vi "SimpleNotifier.vi"() -> ()   [LabVIEW 2014]
panel:
  out "L2":i32
  out "L1":i32
  out "Data 2":dbl(graph)
  out "Data 1":dbl(graph)
  in  "Stop":bool
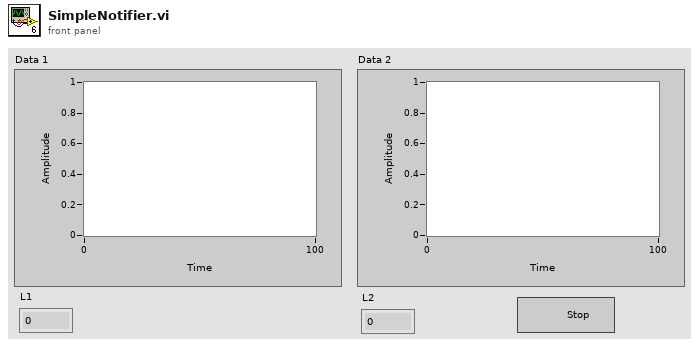
[diagram p1: front panel]
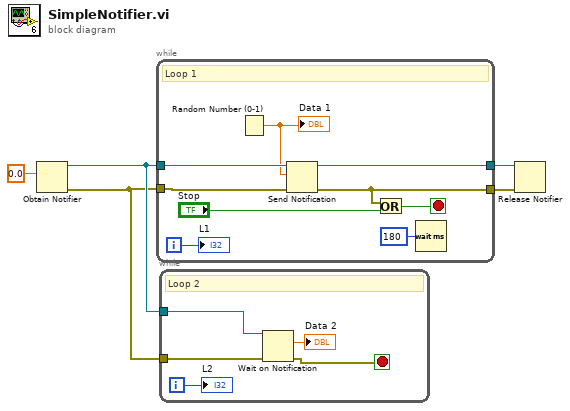
[diagram p0: block diagram]
diagram:
  n1 = Obtain Notifier(notification data type=0.0) -> (notifier out=w2:refnum<notifier>, error out=w1:errorcluster)  [unwired: 3 in, 1 out]
  n2 = while {
    tunnel: w1 -> [w13]
    tunnel: w2 -> [w12]
    tunnel: [w11] -> w3
    tunnel: [w9] -> w4
    i -> [w6]
    stop <- w7 stop-if-true
    # "Loop 1"
    n3 = Random Number (0-1)() -> (number: 0 to 1=w10:dbl)
    "Data 1" <- w10
    n4 = Send Notification(notification=w10, notifier=w12, error in (no error)=w13) -> (notifier out=w11:refnum<notifier>, error out=w9:errorcluster)
    n5 = Or(x=w9, y="Stop") -> (x .or. y?=w7:bool)
    n6 = Wait (ms)(milliseconds to wait=u32 180) -> ()  [unwired: 1 out]
    "L1" <- w6
  }
  n7 = while {
    tunnel: w1 -> [w19]
    tunnel: w2 -> [w18]
    i -> [w15]
    stop <- w16 stop-if-true
    # "Loop 2"
    n8 = Wait on Notification(notifier=w18, error in (no error)=w19) -> (notification=→"Data 2":dbl, error out=w16:errorcluster)  [unwired: 2 in, 2 out]
    "L2" <- w15
  }
  n9 = Release Notifier(notifier=w3, error in (no error)=w4) -> ()  [unwired: 1 in, 3 out]
